vi "rsscope_core_global.vi"() -> ()   [LabVIEW 2018] (continued)
{"Level"=3, "Class Only"=FALSE, "Identifier"="RSSCOPE_ATTR_PROTOCOL_1000BASE_T1_REVERSE_DIFFERENTIAL_SOURCE", "Descriptive Name"="Protocol 1000BASE-T1 Reverse Differential Source", "Data Type"=0, "Command"="BUS{SerialBus}:TBTO:RDIF", "Access"=2, "Range Table"="rsscope_rngProtocolDataSource", "Read Callback"="", "Write Callback"="", "Supported Models"="", "Instrument Options"="K58", "Flags"=0, "Help"="Sets the source of the provided reversed differential signal, if RSSCOPE_ATTR_PROTOCOL_1000BASE_T1_REVERSE_SIGNAL_TYPE is set to differential.\n\nAvailable Repeated Capabilities:\nSerialBus: SB1, SB2, SB3, SB4\r\n\nRemote-control command(s):\nBUS<m>:TBTO:RDIF"}, {"Level"=3, "Class Only"=FALSE, "Identifier"="RSSCOPE_ATTR_PROTOCOL_1000BASE_T1_REVERSE_POSITIVE_SOURCE", "Descriptive Name"="Protocol 1000BASE-T1 Reverse Positive Source", "Data Type"=0, "Command"="BUS{SerialBus}:TBTO:RDAP", "Access"=2, "Range Table"="rsscope_rngProtocolDataSource", "Read Callback"="", "Write Callback"="", "Supported Models"="", "Instrument Options"="K58", "Flags"=0, "Help"="Selects the DA+ source of the provided reversed single ended signal, if RSSCOPE_ATTR_PROTOCOL_1000BASE_T1_REVERSE_SIGNAL_TYPE is set to single.\n\nAvailable Repeated Capabilities:\nSerialBus: SB1, SB2, SB3, SB4\r\n\nRemote-control command(s):\nBUS<m>:TBTO:RDAP"}, {"Level"=3, "Class Only"=FALSE, "Identifier"="RSSCOPE_ATTR_PROTOCOL_1000BASE_T1_REVERSE_NEGATIVE_SOURCE", "Descriptive Name"="Protocol 1000BASE-T1 Reverse Negative Source", "Data Type"=0, "Command"="BUS{SerialBus}:TBTO:RDAM", "Access"=2, "Range Table"="rsscope_rngProtocolDataSource", "Read Callback"="", "Write Callback"="", "Supported Models"="", "Instrument Options"="K58", "Flags"=0, "Help"="Selects the DA- source of the provided reversed single ended signal, if RSSCOPE_ATTR_PROTOCOL_1000BASE_T1_REVERSE_SIGNAL_TYPE is set to single.\n\nAvailable Repeated Capabilities:\nSerialBus: SB1, SB2, SB3, SB4\r\n\nRemote-control command(s):\nBUS<m>:TBTO:RDAM"}, {"Level"=3, "Class Only"=FALSE, "Identifier"="RSSCOPE_ATTR_PROTOCOL_1000BASE_T1_FORWARD_SIGNAL_TYPE", "Descriptive Name"="Protocol 1000BASE-T1 Forward Signal Type", "Data Type"=0, "Command"="BUS{SerialBus}:TBTO:FTYP", "Access"=2, "Range Table"="RsScope_rngSignalType", "Read Callback"="", "Write Callback"="", "Supported Models"="", "Instrument Options"="K58", "Flags"=0, "Help"="Sets the type of forward signal measurement.\n\nAvailable Repeated Capabilities:\nSerialBus: SB1, SB2, SB3, SB4\r\n\nRemote-control command(s):\nBUS<m>:TBTO:FTYP"}, {"Level"=3, "Class Only"=FALSE, "Identifier"="RSSCOPE_ATTR_PROTOCOL_1000BASE_T1_FORWARD_DIFFERENTIAL_SOURCE", "Descriptive Name"="Protocol 1000BASE-T1 Forward Differential Source", "Data Type"=0, "Command"="BUS{SerialBus}:TBTO:FDIF", "Access"=2, "Range Table"="rsscope_rngProtocolDataSource", "Read Callback"="", "Write Callback"="", "Supported Models"="", "Instrument Options"="K58", "Flags"=0, "Help"="Sets the source of the provided forward differential signal, if RSSCOPE_ATTR_PROTOCOL_1000BASE_T1_FORWARD_SIGNAL_TYPE is set to differential.\n\nAvailable Repeated Capabilities:\nSerialBus: SB1, SB2, SB3, SB4\r\n\nRemote-control command(s):\nBUS<m>:TBTO:FDIF"}, {"Level"=3, "Class Only"=FALSE, "Identifier"="RSSCOPE_ATTR_PROTOCOL_1000BASE_T1_FORWARD_POSITIVE_SOURCE", "Descriptive Name"="Protocol 1000BASE-T1 Forward Positive Source", "Data Type"=0, "Command"="BUS{SerialBus}:TBTO:FDAP", "Access"=2, "Range Table"="rsscope_rngProtocolDataSource", "Read Callback"="", "Write Callback"="", "Supported Models"="", "Instrument Options"="K58", "Flags"=0, "Help"="Selects the DA+ source of the provided forward single ended signal, if RSSCOPE_ATTR_PROTOCOL_1000BASE_T1_FORWARD_SIGNAL_TYPE is set to single.\n\nAvailable Repeated Capabilities:\nSerialBus: SB1, SB2, SB3, SB4\r\n\nRemote-control command(s):\nBUS<m>:TBTO:FDAP"}, {"Level"=3, "Class Only"=FALSE, "Identifier"="RSSCOPE_ATTR_PROTOCOL_1000BASE_T1_FORWARD_NEGATIVE_SOURCE", "Descriptive Name"="Protocol 1000BASE-T1 Forward Negative Source", "Data Type"=0, "Command"="BUS{SerialBus}:TBTO:FDAM", "Access"=2, "Range Table"="rsscope_rngProtocolDataSource", "Read Callback"="", "Write Callback"="", "Supported Models"="", "Instrument Options"="K58", "Flags"=0, "Help"="Selects the DA- source of the provided forward single ended signal, if RSSCOPE_ATTR_PROTOCOL_1000BASE_T1_FORWARD_SIGNAL_TYPE is set to single.\n\nAvailable Repeated Capabilities:\nSerialBus: SB1, SB2, SB3, SB4\r\n\nRemote-control command(s):\nBUS<m>:TBTO:FDAM"}, {"Level"=3, "Class Only"=FALSE, "Identifier"="RSSCOPE_ATTR_PROTOCOL_1000BASE_T1_ATTENUATION", "Descriptive Name"="Protocol 1000BASE-T1 Attenuation", "Data Type"=1, "Command"="BUS{SerialBus}:TBTO:ATTN", "Access"=2, "Range Table"="RsScope_rngProtocol1000BASE_T1Attenuation", "Read Callback"="", "Write Callback"="", "Supported Models"="", "Instrument Options"="K58", "Flags"=0, "Help"="Sets the attenuation factor. It is used to de-amplify the reverse signal before subtracting it from the forward signal.\n\nAvailable Repeated Capabilities:\nSerialBus: SB1, SB2, SB3, SB4\r\n\nRemote-control command(s):\nBUS<m>:TBTO:ATTN"}, {"Level"=3, "Class Only"=FALSE, "Identifier"="RSSCOPE_ATTR_PROTOCOL_1000BASE_T1_POLARITY", "Descriptive Name"="Protocol 1000BASE-T1 Polarity", "Data Type"=0, "Command"="BUS{SerialBus}:TBTO:POL", "Access"=2, "Range Table"="rsscope_rngEthernetPolarity", "Read Callback"="", "Write Callback"="", "Supported Models"="", "Instrument Options"="K58", "Flags"=0, "Help"="Selects the polarity of the data signal.\n\nAvailable Repeated Capabilities:\nSerialBus: SB1, SB2, SB3, SB4\r\n\nRemote-control command(s):\nBUS<m>:TBTO:POLarity"}, {"Level"=3, "Class Only"=FALSE, "Identifier"="RSSCOPE_ATTR_PROTOCOL_1000BASE_T1_MODE", "Descriptive Name"="Protocol 1000BASE-T1 Mode", "Data Type"=0, "Command"="BUS{SerialBus}:TBTO:MODE", "Access"=2, "Range Table"="RsScope_rngSignalDirection", "Read Callback"="", "Write Callback"="", "Supported Models"="", "Instrument Options"="K58", "Flags"=0, "Help"="Selects the direction of the full-duplex signal you want to look at.\n\nAvailable Repeated Capabilities:\nSerialBus: SB1, SB2, SB3, SB4\r\n\nRemote-control command(s):\nBUS<m>:TBTO:MODE"}, {"Level"=3, "Class Only"=FALSE, "Identifier"="RSSCOPE_ATTR_PROTOCOL_1000BASE_T1_SYMBOL_RATE", "Descriptive Name"="Protocol 1000BASE-T1 Symbol Rate", "Data Type"=1, "Command"="BUS{SerialBus}:TBTO:SYMR", "Access"=2, "Range Table"="RsScope_rngProtocol1000BASE_T1SymbolRate", "Read Callback"="", "Write Callback"="", "Supported Models"="", "Instrument Options"="K58", "Flags"=0, "Help"="Defines the rate of ternary symbols.\n\nAvailable Repeated Capabilities:\nSerialBus: SB1, SB2, SB3, SB4\r\n\nRemote-control command(s):\nBUS<m>:TBTO:SYMRate"}, {"Level"=3, "Class Only"=TRUE, "Identifier"="", "Descriptive Name"="Decoding Results", "Data Type"=0, "Command"="", "Access"=0, "Range Table"="", "Read Callback"="", "Write Callback"="", "Supported Models"="", "Instrument Options"="", "Flags"=0, "Help"="Returns the 1000BASE-T1 decoding results."}, {"Level"=4, "Class Only"=FALSE, "Identifier"="RSSCOPE_ATTR_PROTOCOL_1000BASE_T1_FRAME_COUNT", "Descriptive Name"="Protocol 1000BASE-T1 Frame Count", "Data Type"=0, "Command"="BUS{SerialBus}:TBTO:RES:FCO?", "Access"=0, "Range Table"="", "Read Callback"="", "Write Callback"="", "Supported Models"="", "Instrument Options"="K58", "Flags"=0, "Help"="Returns the number of decoded frames.\n\nAvailable Repeated Capabilities:\nSerialBus: SB1, SB2, SB3, SB4\r\n\nRemote-control command(s):\nBUS<m>:TBTO:RESult:FCOunt?"}, {"Level"=4, "Class Only"=FALSE, "Identifier"="RSSCOPE_ATTR_PROTOCOL_1000BASE_T1_SELECTED_FRAME", "Descriptive Name"="Protocol 1000BASE-T1 Selected Frame", "Data Type"=0, "Command"="", "Access"=2, "Range Table"="", "Read Callback"="", "Write Callback"="", "Supported Models"="", "Instrument Options"="K58", "Flags"=0, "Help"="Sets the selector for the Frame repeated capability.\n\nAvailable Repeated Capabilities:\nNone\n\nRemote-control command(s):\n"}, {"Level"=4, "Class Only"=FALSE, "Identifier"="RSSCOPE_ATTR_PROTOCOL_1000BASE_T1_FRAME_STATUS", "Descriptive Name"="Protocol 1000BASE-T1 Frame Status", "Data Type"=0, "Command"="BUS{SerialBus}:TBTO:RES:FRAM<Frame>:STAT?", "Access"=0, "Range Table"="RsScope_rngProtocol1000BASE_T1FrameStatus", "Read Callback"="rsscope_Format1000BASE_T1FrameRepCapInt32_ReadCallback.vi", "Write Callback"="", "Supported Models"="", "Instrument Options"="K58", "Flags"=0, "Help"="Returns the state of the frame.\n\nAvailable Repeated Capabilities:\nSerialBus: SB1, SB2, SB3, SB4\r\n\nRemote-control command(s):\nBUS<m>:TBTO:RESult:FRAMe<n>:STATe?"}, {"Level"=4, "Class Only"=FALSE, "Identifier"="RSSCOPE_ATTR_PROTOCOL_1000BASE_T1_FRAME_START_TIME", "Descriptive Name"="Protocol 1000BASE-T1 Frame Start Time", "Data Type"=1, "Command"="BUS{SerialBus}:TBTO:RES:FRAM<Frame>:STAR?", "Access"=0, "Range Table"="", "Read Callback"="rsscope_Format1000BASE_T1FrameRepCapReal64_ReadCallback.vi", "Write Callback"="", "Supported Models"="", "Instrument Options"="K58", "Flags"=0, "Help"="Returns the start time of the selected frame.\n\nAvailable Repeated Capabilities:\nSerialBus: SB1, SB2, SB3, SB4\r\n\nRemote-control command(s):\nBUS<m>:TBTO:RESult:FRAMe<n>:STARt?"}, {"Level"=4, "Class Only"=FALSE, "Identifier"="RSSCOPE_ATTR_PROTOCOL_1000BASE_T1_FRAME_STOP_TIME", "Descriptive Name"="Protocol 1000BASE-T1 Frame Stop Time", "Data Type"=1, "Command"="BUS{SerialBus}:TBTO:RES:FRAM<Frame>:STOP?", "Access"=0, "Range Table"="", "Read Callback"="rsscope_Format1000BASE_T1FrameRepCapReal64_ReadCallback.vi", "Write Callback"="", "Supported Models"="", "Instrument Options"="K58", "Flags"=0, "Help"="Returns the end time of the selected frame.\n\nAvailable Repeated Capabilities:\nSerialBus: SB1, SB2, SB3, SB4\r\n\nRemote-control command(s):\nBUS<m>:TBTO:RESult:FRAMe<n>:STOP?"}, {"Level"=4, "Class Only"=FALSE, "Identifier"="RSSCOPE_ATTR_PROTOCOL_1000BASE_T1_FRAME_LENGTH", "Descriptive Name"="Protocol 1000BASE-T1 Frame Length", "Data Type"=0, "Command"="BUS{SerialBus}:TBTO:RES:FRAM<Frame>:TYPE?", "Access"=0, "Range Table"="", "Read Callback"="rsscope_Format1000BASE_T1FrameRepCapInt32_ReadCallback.vi", "Write Callback"="", "Supported Models"="", "Instrument Options"="K58", "Flags"=0, "Help"="Returns the value of length / type field of the selected frame.\n\nAvailable Repeated Capabilities:\nSerialBus: SB1, SB2, SB3, SB4\r\n\nRemote-control command(s):\nBUS<m>:TBTO:RESult:FRAMe<n>:TYPE?"}, {"Level"=4, "Class Only"=FALSE, "Identifier"="RSSCOPE_ATTR_PROTOCOL_1000BASE_T1_FRAME_CRC", "Descriptive Name"="Protocol 1000BASE-T1 Frame CRC", "Data Type"=5, "Command"="BUS{SerialBus}:TBTO:RES:FRAM<Frame>:CRC?", "Access"=0, "Range Table"="", "Read Callback"="rsscope_Format1000BASE_T1FrameRepCapInt64_ReadCallback.vi", "Write Callback"="", "Supported Models"="", "Instrument Options"="K58", "Flags"=0, "Help"="Returns the CRC (frame check) checksum of the selected frame.\n\nAvailable Repeated Capabilities:\nSerialBus: SB1, SB2, SB3, SB4\r\n\nRemote-control command(s):\nBUS<m>:TBTO:RESult:FRAMe<n>:CRC?"}, {"Level"=4, "Class Only"=FALSE, "Identifier"="RSSCOPE_ATTR_PROTOCOL_1000BASE_T1_FRAME_DATA_BYTES_RAWSTRING", "Descriptive Name"="Protocol 1000BASE-T1 Frame Data Bytes RawString", "Data Type"=6, "Command"="BUS{SerialBus}:TBTO:RES:FRAM<Frame>:DATA?", "Access"=0, "Range Table"="", "Read Callback"="rsscope_Format1000BASE_T1FrameRepCapString_ReadCallback.vi", "Write Callback"="", "Supported Models"="", "Instrument Options"="K58", "Flags"=0, "Help"="Returns the data for the selected frame.\n\nAvailable Repeated Capabilities:\nSerialBus: SB1, SB2, SB3, SB4\r\n\nRemote-control command(s):\nBUS<m>:TBTO:RESult:FRAMe<n>:DATA?"}, {"Level"=4, "Class Only"=FALSE, "Identifier"="RSSCOPE_ATTR_PROTOCOL_1000BASE_T1_FRAME_DESTINATION", "Descriptive Name"="Protocol 1000BASE-T1 Frame Destination", "Data Type"=2, "Command"="BUS{SerialBus}:TBTO:RES:FRAM<Frame>:DEST?", "Access"=0, "Range Table"="", "Read Callback"="rsscope_Format1000BASE_T1FrameRepCapString_ReadCallback.vi", "Write Callback"="", "Supported Models"="", "Instrument Options"="K58", "Flags"=0, "Help"="Returns the destination address of the selected frame.\n\nAvailable Repeated Capabilities:\nSerialBus: SB1, SB2, SB3, SB4\r\n\nRemote-control command(s):\nBUS<m>:TBTO:RESult:FRAMe<n>:DESTaddress?"}, {"Level"=4, "Class Only"=FALSE, "Identifier"="RSSCOPE_ATTR_PROTOCOL_1000BASE_T1_FRAME_DESTINATION_SYMBOLS", "Descriptive Name"="Protocol 1000BASE-T1 Frame Destination Symbols", "Data Type"=2, "Command"="BUS{SerialBus}:TBTO:RES:FRAM<Frame>:DSYM?", "Access"=0, "Range Table"="", "Read Callback"="rsscope_Format1000BASE_T1FrameRepCapString_ReadCallback.vi", "Write Callback"="", "Supported Models"="", "Instrument Options"="K58", "Flags"=0, "Help"="Returns the destination symbols of the selected frame.\n\nAvailable Repeated Capabilities:\nSerialBus: SB1, SB2, SB3, SB4\r\n\nRemote-control command(s):\nBUS<m>:TBTO:RESult:FRAMe<n>:DSYMbol?"}, {"Level"=4, "Class Only"=FALSE, "Identifier"="RSSCOPE_ATTR_PROTOCOL_1000BASE_T1_FRAME_SOURCE", "Descriptive Name"="Protocol 1000BASE-T1 Frame Source", "Data Type"=2, "Command"="BUS{SerialBus}:TBTO:RES:FRAM<Frame>:SRC?", "Access"=0, "Range Table"="", "Read Callback"="rsscope_Format1000BASE_T1FrameRepCapString_ReadCallback.vi", "Write Callback"="", "Supported Models"="", "Instrument Options"="K58", "Flags"=0, "Help"="Returns the source address of the selected frame.\n\nAvailable Repeated Capabilities:\nSerialBus: SB1, SB2, SB3, SB4\r\n\nRemote-control command(s):\nBUS<m>:TBTO:RESult:FRAMe<n>:SRCaddress?"}, {"Level"=4, "Class Only"=FALSE, "Identifier"="RSSCOPE_ATTR_PROTOCOL_1000BASE_T1_FRAME_SOURCE_SYMBOLS", "Descriptive Name"="Protocol 1000BASE-T1 Frame Source Symbols", "Data Type"=2, "Command"="BUS{SerialBus}:TBTO:RES:FRAM<Frame>:SSYM?", "Access"=0, "Range Table"="", "Read Callback"="rsscope_Format1000BASE_T1FrameRepCapString_ReadCallback.vi", "Write Callback"="", "Supported Models"="", "Instrument Options"="K58", "Flags"=0, "Help"="Returns the source symbols of the selected frame.\n\nAvailable Repeated Capabilities:\nSerialBus: SB1, SB2, SB3, SB4\r\n\nRemote-control command(s):\nBUS<m>:TBTO:RESult:FRAMe<n>:SSYMbol?"}, {"Level"=4, "Class Only"=FALSE, "Identifier"="RSSCOPE_ATTR_PROTOCOL_1000BASE_T1_FRAME_BIT_RATE", "Descriptive Name"="Protocol 1000BASE-T1 Frame Bit Rate", "Data Type"=5, "Command"="BUS{SerialBus}:TBTO:RES:FRAM<Frame>:BITR?", "Access"=0, "Range Table"="", "Read Callback"="rsscope_Format1000BASE_T1FrameRepCapInt64_ReadCallback.vi", "Write Callback"="", "Supported Models"="", "Instrument Options"="K58", "Flags"=0, "Help"="Returns the primary bit rate.\n\nAvailable Repeated Capabilities:\nSerialBus: SB1, SB2, SB3, SB4\r\n\nRemote-control command(s):\nBUS<m>:TBTO:RESult:FRAMe<n>:BITRate?"}, {"Level"=4, "Class Only"=FALSE, "Identifier"="RSSCOPE_ATTR_PROTOCOL_1000BASE_T1_FRAME_TYPE", "Descriptive Name"="Protocol 1000BASE-T1 Frame Type", "Data Type"=0, "Command"="BUS{SerialBus}:TBTO:RES:FRAM<Frame>:FTYP?", "Access"=0, "Range Table"="RsScope_rngProtocol1000BASE_T1FrameType", "Read Callback"="rsscope_Format1000BASE_T1FrameRepCapInt32_ReadCallback.vi", "Write Callback"="", "Supported Models"="", "Instrument Options"="K58", "Flags"=0, "Help"="Returns the type of the selected frame.\n\nAvailable Repeated Capabilities:\nSerialBus: SB1, SB2, SB3, SB4\r\n\nRemote-control command(s):\nBUS<m>:TBTO:RESult:FRAMe<n>:FTYPe?"}, {"Level"=4, "Class Only"=FALSE, "Identifier"="RSSCOPE_ATTR_PROTOCOL_1000BASE_T1_FRAME_NUMBER_OF_WORDS", "Descriptive Name"="Protocol 1000BASE-T1 Frame Number Of Words", "Data Type"=5, "Command"="BUS{SerialBus}:TBTO:RES:FRAM<Frame>:NUMW?", "Access"=0, "Range Table"="", "Read Callback"="rsscope_Format1000BASE_T1FrameRepCapInt64_ReadCallback.vi", "Write Callback"="", "Supported Models"="", "Instrument Options"="K58", "Flags"=0, "Help"="Returns the number of decoded words for the selected frame.\n\nAvailable Repeated Capabilities:\nSerialBus: SB1, SB2, SB3, SB4\r\n\nRemote-control command(s):\nBUS<m>:TBTO:RESult:FRAMe<n>:NUMWords?"}, {"Level"=4, "Class Only"=FALSE, "Identifier"="RSSCOPE_ATTR_PROTOCOL_1000BASE_T1_SELECTED_WORD", "Descriptive Name"="Protocol 1000BASE-T1 Selected Word", "Data Type"=5, "Command"="", "Access"=2, "Range Table"="", "Read Callback"="", "Write Callback"="", "Supported Models"="", "Instrument Options"="K58", "Flags"=0, "Help"="Sets the selector for the Word repeated capability.\n\nAvailable Repeated Capabilities:\nNone\n\nRemote-control command(s):\n"}, {"Level"=4, "Class Only"=FALSE, "Identifier"="RSSCOPE_ATTR_PROTOCOL_1000BASE_T1_FRAME_WORD_TYPE", "Descriptive Name"="Protocol 1000BASE-T1 Frame Word Type", "Data Type"=2, "Command"="BUS{SerialBus}:TBTO:RES:FRAM<Frame>:WORD<Word>:TYPE?", "Access"=0, "Range Table"="", "Read Callback"="rsscope_Format1000BASE_T1WordRepCapString_ReadCallback.vi", "Write Callback"="", "Supported Models"="", "Instrument Options"="K58", "Flags"=0, "Help"="Returns the data type for the selected word.\n\nAvailable Repeated Capabilities:\nSerialBus: SB1, SB2, SB3, SB4\r\n\nRemote-control command(s):\nBUS<m>:TBTO:RESult:FRAMe<n>:WORD<o>:TYPE?"}, {"Level"=4, "Class Only"=FALSE, "Identifier"="RSSCOPE_ATTR_PROTOCOL_1000BASE_T1_FRAME_WORD_VALUE", "Descriptive Name"="Protocol 1000BASE-T1 Frame Word Value", "Data Type"=0, "Command"="BUS{SerialBus}:TBTO:RES:FRAM<Frame>:WORD<Word>:VAL?", "Access"=0, "Range Table"="", "Read Callback"="rsscope_Format1000BASE_T1WordRepCapInt32_ReadCallback.vi", "Write Callback"="", "Supported Models"="", "Instrument Options"="K58", "Flags"=0, "Help"="Returns the data value for the selected word.\n\nAvailable Repeated Capabilities:\nSerialBus: SB1, SB2, SB3, SB4\r\n\nRemote-control command(s):\nBUS<m>:TBTO:RESult:FRAMe<n>:WORD<o>:VALue?"}, {"Level"=1, "Class Only"=TRUE, "Identifier"="", "Descriptive Name"="Power Analysis", "Data Type"=0, "Command"="", "Access"=0, "Range Table"="", "Read Callback"="", "Write Callback"="", "Supported Models"="", "Instrument Options"="", "Flags"=0, "Help"="Power Analysis"}, {"Level"=2, "Class Only"=FALSE, "Identifier"="RSSCOPE_ATTR_POWER_ANALYSIS_MODE", "Descriptive Name"="Power Analysis Mode", "Data Type"=4, "Command"="POW:ENAB", "Access"=1, "Range Table"="", "Read Callback"="", "Write Callback"="", "Supported Models"="", "Instrument Options"="", "Flags"=0, "Help"="Activates the power analysis measurement.\n\nAvailable Repeated Capabilities:\nNone\n\nRemote-control command(s):\nPOWer:ENABle"}, {"Level"=2, "Class Only"=TRUE, "Identifier"="", "Descriptive Name"="Source", "Data Type"=0, "Command"="", "Access"=0, "Range Table"="", "Read Callback"="", "Write Callback"="", "Supported Models"="", "Instrument Options"="", "Flags"=0, "Help"="Class for attributes with SourceNumber repcap."}, {"Level"=3, "Class Only"=FALSE, "Identifier"="RSSCOPE_ATTR_POWER_ANALYSIS_VOLTAGE_SOURCE", "Descriptive Name"="Power Analysis Voltage Source", "Data Type"=0, "Command"="POW:SOUR:VOLT{SourceNumber}", "Access"=2, "Range Table"="RsScope_rngPowerAnalysisSource", "Read Callback"="", "Write Callback"="", "Supported Models"="", "Instrument Options"="", "Flags"=0, "Help"="Sets the channel for the voltage source input.\n\nAvailable Repeated Capabilities:\nSourceNumber: SN1, SN2, SN3, SN4\r\n\nRemote-control command(s):\nPOWer:SOURce:VOLTage<1..4>"}, {"Level"=3, "Class Only"=FALSE, "Identifier"="RSSCOPE_ATTR_POWER_ANALYSIS_CURRENT_SOURCE", "Descriptive Name"="Power Analysis Current Source", "Data Type"=0, "Command"="POW:SOUR:CURR{SourceNumber}", "Access"=2, "Range Table"="RsScope_rngPowerAnalysisSource", "Read Callback"="", "Write Callback"="", "Supported Models"="", "Instrument Options"="", "Flags"=0, "Help"="Sets the channel for the current source input.\n\nAvailable Repeated Capabilities:\nSourceNumber: SN1, SN2, SN3, SN4\r\n\nRemote-control command(s):\nPOWer:SOURce:CURRent<1..2>"}, {"Level"=2, "Class Only"=TRUE, "Identifier"="", "Descriptive Name"="Deskew", "Data Type"=0, "Command"="", "Access"=0, "Range Table"="", "Read Callback"="", "Write Callback"="", "Supported Models"="", "Instrument Options"="", "Flags"=0, "Help"="Deskew of the current and voltage probes"}, {"Level"=3, "Class Only"=FALSE, "Identifier"="RSSCOPE_ATTR_POWER_ANALYSIS_START_DESKEW", "Descriptive Name"="Power Analysis Start Deskew", "Data Type"=4, "Command"="POW:DESK:EXEC;*WAI", "Access"=1, "Range Table"="", "Read Callback"="", "Write Callback"="", "Supported Models"="", "Instrument Options"="", "Flags"=0, "Help"="Starts the auto deskew.\n\nAvailable Repeated Capabilities:\nNone\n\nRemote-control command(s):\nPOWer:DESKew:EXECute"}, {"Level"=3, "Class Only"=FALSE, "Identifier"="RSSCOPE_ATTR_POWER_ANALYSIS_DESKEW_RESET", "Descriptive Name"="Power Analysis Deskew Reset", "Data Type"=3, "Command"="POW:DESK:RES", "Access"=2, "Range Table"="", "Read Callback"="", "Write Callback"="", "Supported Models"="", "Instrument Options"="", "Flags"=0, "Help"="Overwrites the present skew setup.\n\nAvailable Repeated Capabilities:\nNone\n\nRemote-control command(s):\nPOWer:DESKew:RESet"}, {"Level"=3, "Class Only"=FALSE, "Identifier"="RSSCOPE_ATTR_POWER_ANALYSIS_DESKEW_TIME", "Descriptive Name"="Power Analysis Deskew Time", "Data Type"=1, "Command"="POW:DESK:TIME?", "Access"=0, "Range Table"="", "Read Callback"="", "Write Callback"="", "Supported Models"="", "Instrument Options"="", "Flags"=0, "Help"="Queries the result of the auto deskew.\n\nAvailable Repeated Capabilities:\nNone\n\nRemote-control command(s):\nPOWer:DESKew:TIME?"}, {"Level"=3, "Class Only"=FALSE, "Identifier"="RSSCOPE_ATTR_POWER_ANALYSIS_DESKEW_CURRENT", "Descriptive Name"="Power Analysis Deskew Current", "Data Type"=4, "Command"="POW:DESK:CURR", "Access"=1, "Range Table"="", "Read Callback"="", "Write Callback"="", "Supported Models"="", "Instrument Options"="", "Flags"=0, "Help"="Applies the result of the auto deskew to the &apos;Skew offset&apos; value.\n\nAvailable Repeated Capabilities:\nNone\n\nRemote-control command(s):\nPOWer:DESKew:CURRent"}, {"Level"=3, "Class Only"=FALSE, "Identifier"="RSSCOPE_ATTR_POWER_ANALYSIS_DESKEW_USER_DEFINED_RESET", "Descriptive Name"="Power Analysis Deskew User Defined Reset", "Data Type"=3, "Command"="POW:DESK:UDPR", "Access"=2, "Range Table"="", "Read Callback"="", "Write Callback"="", "Supported Models"="", "Instrument Options"="", "Flags"=0, "Help"="Activates or deactivates a user defined setup. If ON, the instrument setup including probe setup and the deskew values are written to a user defined preset file (saveset) that can be loaded using MMEMory:RCL\n\nAvailable Repeated Capabilities:\nNone\n\nRemote-control command(s):\nPOWer:DESKew:UDPReset"}, {"Level"=3, "Class Only"=TRUE, "Identifier"="", "Descriptive Name"="Channel", "Data Type"=0, "Command"="", "Access"=0, "Range Table"="", "Read Callback"="", "Write Callback"="", "Supported Models"="", "Instrument Options"="", "Flags"=0, "Help"="Commands depended on channel number (repeated capability Channel)"}, {"Level"=4, "Class Only"=FALSE, "Identifier"="RSSCOPE_ATTR_POWER_ANALYSE_PROBE_MODE", "Descriptive Name"="Power Analyse Probe Mode", "Data Type"=0, "Command"="PROB{Channel}:SET:DISP", "Access"=2, "Range Table"="RsScope_rngPowerAnalyseProbeMode", "Read Callback"="", "Write Callback"="", "Supported Models"="", "Instrument Options"="", "Flags"=0, "Help"="Selects the input voltages to be measured by the Probe Meter of an R&S differential active probe.\n\nAvailable Repeated Capabilities:\nChannel: CH1, CH2, CH3, CH4, CHExt\r\n\nRemote-control command(s):\nPROBe<m>:SETup:DISPlaydiff"}, {"Level"=2, "Class Only"=TRUE, "Identifier"="", "Descriptive Name"="DUT", "Data Type"=0, "Command"="", "Access"=0, "Range Table"="", "Read Callback"="", "Write Callback"="", "Supported Models"="", "Instrument Options"="", "Flags"=0, "Help"="Characterizes your device under test (DUT)."}, {"Level"=3, "Class Only"=FALSE, "Identifier"="RSSCOPE_ATTR_POWER_ANALYSIS_DUT_NAME", "Descriptive Name"="Power Analysis DUT Name", "Data Type"=2, "Command"="POW:REP:DUT", "Access"=2, "Range Table"="", "Read Callback"="", "Write Callback"="", "Supported Models"="", "Instrument Options"="", "Flags"=0, "Help"="Enter a name for your DUT.\n\nAvailable Repeated Capabilities:\nNone\n\nRemote-control command(s):\nPOWer:REPort:DUT"}, {"Level"=3, "Class Only"=FALSE, "Identifier"="RSSCOPE_ATTR_POWER_ANALYSIS_USER", "Descriptive Name"="Power Analysis User", "Data Type"=2, "Command"="POW:REP:USER", "Access"=2, "Range Table"="", "Read Callback"="", "Write Callback"="", "Supported Models"="", "Instrument Options"="", "Flags"=0, "Help"="Enter a user.\n\nAvailable Repeated Capabilities:\nNone\n\nRemote-control command(s):\nPOWer:REPort:USER"}, {"Level"=3, "Class Only"=FALSE, "Identifier"="RSSCOPE_ATTR_POWER_ANALYSIS_SITE", "Descriptive Name"="Power Analysis Site", "Data Type"=2, "Command"="POW:REP:SITE", "Access"=2, "Range Table"="", "Read Callback"="", "Write Callback"="", "Supported Models"="", "Instrument Options"="", "Flags"=0, "Help"="Enter a site.\n\nAvailable Repeated Capabilities:\nNone\n\nRemote-control command(s):\nPOWer:REPort:SITE"}, {"Level"=3, "Class Only"=FALSE, "Identifier"="RSSCOPE_ATTR_POWER_ANALYSIS_TEMPERATURE", "Descriptive Name"="Power Analysis Temperature", "Data Type"=0, "Command"="POW:REP:TEMP", "Access"=2, "Range Table"="", "Read Callback"="", "Write Callback"="", "Supported Models"="", "Instrument Options"="", "Flags"=0, "Help"="Enter a temperature.\n\nAvailable Repeated Capabilities:\nNone\n\nRemote-control command(s):\nPOWer:REPort:TEMPerature"}, {"Level"=3, "Class Only"=FALSE, "Identifier"="RSSCOPE_ATTR_POWER_ANALYSIS_DESCRIPTION", "Descriptive Name"="Power Analysis Description", "Data Type"=2, "Command"="POW:REP:DESC", "Access"=2, "Range Table"="", "Read Callback"="", "Write Callback"="", "Supported Models"="", "Instrument Options"="", "Flags"=0, "Help"="Enter a description.\n\nAvailable Repeated Capabilities:\nNone\n\nRemote-control command(s):\nPOWer:REPort:DESCription"}, {"Level"=2, "Class Only"=TRUE, "Identifier"="", "Descriptive Name"="Report", "Data Type"=0, "Command"="", "Access"=0, "Range Table"="", "Read Callback"="", "Write Callback"="", "Supported Models"="", "Instrument Options"="", "Flags"=0, "Help"="Power Measurement Reports"}, {"Level"=3, "Class Only"=FALSE, "Identifier"="RSSCOPE_ATTR_POWER_ANALYSIS_REPORT_ADD", "Descriptive Name"="Power Analysis Report Add", "Data Type"=0, "Command"="POW:REP:TEST:ADD", "Access"=1, "Range Table"="RsScope_rngPowerAnalysisMeasurementType", "Read Callback"="", "Write Callback"="", "Supported Models"="", "Instrument Options"="", "Flags"=0, "Help"="Adds the selected measurement to the report.\n\nAvailable Repeated Capabilities:\nNone\n\nRemote-control command(s):\nPOWer:REPort:TEST:ADD"}, {"Level"=3, "Class Only"=FALSE, "Identifier"="RSSCOPE_ATTR_POWER_ANALYSIS_REPORT_SEL_ALL", "Descriptive Name"="Power Analysis Report Select All", "Data Type"=0, "Command"="POW:REP:TEST:SEA", "Access"=1, "Range Table"="RsScope_rngPowerAnalysisMeasurementType", "Read Callback"="", "Write Callback"="", "Supported Models"="", "Instrument Options"="", "Flags"=0, "Help"="Selects all result reports.\n\nAvailable Repeated Capabilities:\nNone\n\nRemote-control command(s):\nPOWer:REPort:TEST:SEA"}, {"Level"=3, "Class Only"=FALSE, "Identifier"="RSSCOPE_ATTR_POWER_ANALYSIS_REPORT_SEL_NONE", "Descriptive Name"="Power Analysis Report Deselect All", "Data Type"=0, "Command"="POW:REP:TEST:DSEA", "Access"=1, "Range Table"="RsScope_rngPowerAnalysisMeasurementType", "Read Callback"="", "Write Callback"="", "Supported Models"="", "Instrument Options"="", "Flags"=0, "Help"="Deselects all result reports.\n\nAvailable Repeated Capabilities:\nNone\n\nRemote-control command(s):\nPOWer:REPort:TEST:DSEA"}, {"Level"=3, "Class Only"=FALSE, "Identifier"="RSSCOPE_ATTR_POWER_ANALYSIS_REPORT_SEL_REMOVE", "Descriptive Name"="Power Analysis Report Remove Selected", "Data Type"=0, "Command"="POW:REP:TEST:RSE", "Access"=1, "Range Table"="RsScope_rngPowerAnalysisMeasurementType", "Read Callback"="", "Write Callback"="", "Supported Models"="", "Instrument Options"="", "Flags"=0, "Help"="Removes the selected result report.\n\nAvailable Repeated Capabilities:\nNone\n\nRemote-control command(s):\nPOWer:REPort:TEST:RSE"}, {"Level"=3, "Class Only"=FALSE, "Identifier"="RSSCOPE_ATTR_POWER_ANALYSIS_REPORT_SEL_INVERT", "Descriptive Name"="Power Analysis Report Invert Selection", "Data Type"=0, "Command"="POW:REP:TEST:ISE", "Access"=1, "Range Table"="RsScope_rngPowerAnalysisMeasurementType", "Read Callback"="", "Write Callback"="", "Supported Models"="", "Instrument Options"="", "Flags"=0, "Help"="Inverts the selection of all result reports, meaning that all selected result reports are deselected and vice versa.\n\nAvailable Repeated Capabilities:\nNone\n\nRemote-control command(s):\nPOWer:REPort:TEST:ISE"}, {"Level"=3, "Class Only"=FALSE, "Identifier"="RSSCOPE_ATTR_POWER_ANALYSIS_REPORT_FILE_NEW", "Descriptive Name"="Power Analysis Report File New", "Data Type"=4, "Command"="POW:REP:FILE:NEW", "Access"=1, "Range Table"="", "Read Callback"="", "Write Callback"="", "Supported Models"="", "Instrument Options"="", "Flags"=0, "Help"="Creates new file.\n\nAvailable Repeated Capabilities:\nNone\n\nRemote-control command(s):\nPOWer:REPort:FILE:NEW"}, {"Level"=3, "Class Only"=FALSE, "Identifier"="RSSCOPE_ATTR_POWER_ANALYSIS_REPORT_FILE_NAME", "Descriptive Name"="Power Analysis Report File Name", "Data Type"=2, "Command"="POW:REP:FILE:NAME", "Access"=1, "Range Table"="", "Read Callback"="", "Write Callback"="", "Supported Models"="", "Instrument Options"="", "Flags"=0, "Help"="Renames the file\n\nAvailable Repeated Capabilities:\nNone\n\nRemote-control command(s):\nPOWer:REPort:FILE:NAME"}, {"Level"=3, "Class Only"=FALSE, "Identifier"="RSSCOPE_ATTR_POWER_ANALYSIS_REPORT_FILE_SAVE", "Descriptive Name"="Power Analysis Report File Save", "Data Type"=4, "Command"="POW:REP:FILE:SAVE", "Access"=1, "Range Table"="", "Read Callback"="", "Write Callback"="", "Supported Models"="", "Instrument Options"="", "Flags"=0, "Help"="Saves the file\n\nAvailable Repeated Capabilities:\nNone\n\nRemote-control command(s):\nPOWer:REPort:FILE:SAVE"}, {"Level"=3, "Class Only"=FALSE, "Identifier"="RSSCOPE_ATTR_POWER_ANALYSIS_REPORT_FILE_DELETE", "Descriptive Name"="Power Analysis Report File Delete", "Data Type"=4, "Command"="POW:REP:FILE:DEL", "Access"=1, "Range Table"="", "Read Callback"="", "Write Callback"="", "Supported Models"="", "Instrument Options"="", "Flags"=0, "Help"="Deletes the selected file\n\nAvailable Repeated Capabilities:\nNone\n\nRemote-control command(s):\nPOWer:REPort:FILE:DELete"}, {"Level"=3, "Class Only"=TRUE, "Identifier"="", "Descriptive Name"="Layout", "Data Type"=0, "Command"="", "Access"=0, "Range Table"="", "Read Callback"="", "Write Callback"="", "Supported Models"="", "Instrument Options"="", "Flags"=0, "Help"="Sets a layout for your report."}, {"Level"=4, "Class Only"=FALSE, "Identifier"="RSSCOPE_ATTR_POWER_ANALYSIS_REPORT_PAPER_SIZE", "Descriptive Name"="Power Analysis Report Paper Size", "Data Type"=0, "Command"="POW:REP:PAP", "Access"=2, "Range Table"="RsScope_rngPowerAnalysisReportPaperSize", "Read Callback"="", "Write Callback"="", "Supported Models"="", "Instrument Options"="", "Flags"=0, "Help"="Sets the paper size.\n\nAvailable Repeated Capabilities:\nNone\n\nRemote-control command(s):\nPOWer:REPort:PAPersize"}, {"Level"=4, "Class Only"=FALSE, "Identifier"="RSSCOPE_ATTR_POWER_ANALYSIS_REPORT_FONT", "Descriptive Name"="Power Analysis Report Font", "Data Type"=0, "Command"="POW:REP:FONT:FAMI", "Access"=2, "Range Table"="RsScope_rngPowerAnalysisReportFont", "Read Callback"="", "Write Callback"="", "Supported Models"="", "Instrument Options"="", "Flags"=0, "Help"="Selects the font family.\n\nAvailable Repeated Capabilities:\nNone\n\nRemote-control command(s):\nPOWer:REPort:FONT:FAMI"}, {"Level"=4, "Class Only"=FALSE, "Identifier"="RSSCOPE_ATTR_POWER_ANALYSIS_REPORT_FONT_SIZE", "Descriptive Name"="Power Analysis Report Font Size", "Data Type"=0, "Command"="POW:REP:FONT:SIZE", "Access"=2, "Range Table"="RsScope_rngPowerAnalysisReportFontSize", "Read Callback"="", "Write Callback"="", "Supported Models"="", "Instrument Options"="", "Flags"=0, "Help"="Selects the font size.\n\nAvailable Repeated Capabilities:\nNone\n\nRemote-control command(s):\nPOWer:REPort:FONT:SIZE"}, {"Level"=4, "Class Only"=FALSE, "Identifier"="RSSCOPE_ATTR_POWER_ANALYSIS_REPORT_FONT_COLOR", "Descriptive Name"="Power Analysis Report Font Color", "Data Type"=0, "Command"="POW:REP:FONT:COLO", "Access"=2, "Range Table"="", "Read Callback"="", "Write Callback"="", "Supported Models"="", "Instrument Options"="", "Flags"=0, "Help"="Selects the font color.\n\nAvailable Repeated Capabilities:\nNone\n\nRemote-control command(s):\nPOWer:REPort:FONT:COLO"}, {"Level"=4, "Class Only"=FALSE, "Identifier"="RSSCOPE_ATTR_POWER_ANALYSIS_REPORT_LOGO", "Descriptive Name"="Power Analysis Report Logo", "Data Type"=2, "Command"="POW:REP:LOGO", "Access"=2, "Range Table"="", "Read Callback"="", "Write Callback"="", "Supported Models"="", "Instrument Options"="", "Flags"=0, "Help"="Selects a path to a logo picture file.\n\nAvailable Repeated Capabilities:\nNone\n\nRemote-control command(s):\nPOWer:REPort:LOGO"}, {"Level"=4, "Class Only"=FALSE, "Identifier"="RSSCOPE_ATTR_POWER_ANALYSIS_REPORT_INV_COLOR", "Descriptive Name"="Power Analysis Report Invert Scr Color", "Data Type"=3, "Command"="POW:REP:INV", "Access"=2, "Range Table"="", "Read Callback"="", "Write Callback"="", "Supported Models"="", "Instrument Options"="", "Flags"=0, "Help"="Inverts the screenshot colors.\n\nAvailable Repeated Capabilities:\nNone\n\nRemote-control command(s):\nPOWer:REPort:INVert"}, {"Level"=3, "Class Only"=TRUE, "Identifier"="", "Descriptive Name"="Content", "Data Type"=0, "Command"="", "Access"=0, "Range Table"="", "Read Callback"="", "Write Callback"="", "Supported Models"="", "Instrument Options"="", "Flags"=0, "Help"="Defines the content of report."}, {"Level"=4, "Class Only"=FALSE, "Identifier"="RSSCOPE_ATTR_POWER_ANALYSIS_REPORT_CONTENT_TITLE", "Descriptive Name"="Power Analysis Report Content Title", "Data Type"=3, "Command"="POW:REP:CONT:TITL", "Access"=2, "Range Table"="", "Read Callback"="", "Write Callback"="", "Supported Models"="", "Instrument Options"="", "Flags"=0, "Help"="Adds a Title page to the report. The contents can be set up in the &apos;DUT&apos;\n\nAvailable Repeated Capabilities:\nNone\n\nRemote-control command(s):\nPOWer:REPort:CONTent:TITLe"}, {"Level"=4, "Class Only"=FALSE, "Identifier"="RSSCOPE_ATTR_POWER_ANALYSIS_REPORT_CONTENT_MSETUP", "Descriptive Name"="Power Analysis Report Content Measurement Setup", "Data Type"=0, "Command"="POW:REP:CONT:MSET", "Access"=2, "Range Table"="RsScope_rngPowerAnalysisReportContentSetup", "Read Callback"="", "Write Callback"="", "Supported Models"="", "Instrument Options"="", "Flags"=0, "Help"="Adds a graphic of the measurement setup.\n\nAvailable Repeated Capabilities:\nNone\n\nRemote-control command(s):\nPOWer:REPort:CONTent:MSETup"}, {"Level"=4, "Class Only"=FALSE, "Identifier"="RSSCOPE_ATTR_POWER_ANALYSIS_REPORT_CONTENT_SETTINGS", "Descriptive Name"="Power Analysis Report Content Settings", "Data Type"=0, "Command"="POW:REP:CONT:SETT", "Access"=2, "Range Table"="RsScope_rngPowerAnalysisReportContentSetup", "Read Callback"="", "Write Callback"="", "Supported Models"="", "Instrument Options"="", "Flags"=0, "Help"="Adds the settings of the analysis.\n\nAvailable Repeated Capabilities:\nNone\n\nRemote-control command(s):\nPOWer:REPort:CONTent:SETTings"}, {"Level"=4, "Class Only"=FALSE, "Identifier"="RSSCOPE_ATTR_POWER_ANALYSIS_REPORT_CONTENT_VSETUP", "Descriptive Name"="Power Analysis Report Content Vertical Setup", "Data Type"=0, "Command"="POW:REP:CONT:VSET", "Access"=2, "Range Table"="RsScope_rngPowerAnalysisReportContentSetup", "Read Callback"="", "Write Callback"="", "Supported Models"="", "Instrument Options"="", "Flags"=0, "Help"="Adds the vertical setup settings.\n\nAvailable Repeated Capabilities:\nNone\n\nRemote-control command(s):\nPOWer:REPort:CONTent:VSETup"}, {"Level"=4, "Class Only"=FALSE, "Identifier"="RSSCOPE_ATTR_POWER_ANALYSIS_REPORT_CONTENT_HSETUP", "Descriptive Name"="Power Analysis Report Content Horizontal Setup", "Data Type"=0, "Command"="POW:REP:CONT:HSET", "Access"=2, "Range Table"="RsScope_rngPowerAnalysisReportContentSetup", "Read Callback"="", "Write Callback"="", "Supported Models"="", "Instrument Options"="", "Flags"=0, "Help"="Adds the horizontal setup settings.\n\nAvailable Repeated Capabilities:\nNone\n\nRemote-control command(s):\nPOWer:REPort:CONTent:HSETup"}, {"Level"=4, "Class Only"=FALSE, "Identifier"="RSSCOPE_ATTR_POWER_ANALYSIS_REPORT_CONTENT_TSETUP", "Descriptive Name"="Power Analysis Report Content Trigger Setup", "Data Type"=0, "Command"="POW:REP:CONT:TSET", "Access"=2, "Range Table"="RsScope_rngPowerAnalysisReportContentSetup", "Read Callback"="", "Write Callback"="", "Supported Models"="", "Instrument Options"="", "Flags"=0, "Help"="Adds the trigger setup settings.\n\nAvailable Repeated Capabilities:\nNone\n\nRemote-control command(s):\nPOWer:REPort:CONTent:TSETup"}, {"Level"=4, "Class Only"=FALSE, "Identifier"="RSSCOPE_ATTR_POWER_ANALYSIS_REPORT_CONTENT_MEAS", "Descriptive Name"="Power Analysis Report Content Measured Signal", "Data Type"=0, "Command"="POW:REP:CONT:MSIG", "Access"=2, "Range Table"="RsScope_rngPowerAnalysisReportContentSetup", "Read Callback"="", "Write Callback"="", "Supported Models"="", "Instrument Options"="", "Flags"=0, "Help"="Adds a diagram of the measured signal.\n\nAvailable Repeated Capabilities:\nNone\n\nRemote-control command(s):\nPOWer:REPort:CONTent:MSIGnal"}, {"Level"=4, "Class Only"=FALSE, "Identifier"="RSSCOPE_ATTR_POWER_ANALYSIS_REPORT_CONTENT_RESULTS", "Descriptive Name"="Power Analysis Report Content Results", "Data Type"=0, "Command"="POW:REP:CONT:RESU", "Access"=2, "Range Table"="RsScope_rngPowerAnalysisReportContentSetup", "Read Callback"="", "Write Callback"="", "Supported Models"="", "Instrument Options"="", "Flags"=0, "Help"="Adds the result box.\n\nAvailable Repeated Capabilities:\nNone\n\nRemote-control command(s):\nPOWer:REPort:CONTent:RESU"}, {"Level"=2, "Class Only"=TRUE, "Identifier"="", "Descriptive Name"="Power Quality", "Data Type"=0, "Command"="", "Access"=0, "Range Table"="", "Read Callback"="", "Write Callback"="", "Supported Models"="", "Instrument Options"="", "Flags"=0, "Help"="The &apos;Power Quality&apos; analysis measurements include the real power, the reactive power and the apparent power as well as the power factor. The crest factors and the phase angle between the current and voltage are also measured. These properties describe the power transfer in the system and allow you to characterize the power quality of the system."}, {"Level"=3, "Class Only"=FALSE, "Identifier"="RSSCOPE_ATTR_START_POWER_QUALITY_MEASUREMENT", "Descriptive Name"="Start Power Quality Measurement", "Data Type"=4, "Command"="POW:QUAL:EXEC", "Access"=1, "Range Table"="", "Read Callback"="", "Write Callback"="", "Supported Models"="", "Instrument Options"="", "Flags"=0, "Help"="Starts the power quality measurement.\n\nAvailable Repeated Capabilities:\nNone\n\nRemote-control command(s):\nPOWer:QUALity:EXECute"}, {"Level"=3, "Class Only"=FALSE, "Identifier"="RSSCOPE_ATTR_POWER_QUALITY_FREQUENCY", "Descriptive Name"="Power Quality Frequency", "Data Type"=0, "Command"="POW:QUAL:FREQ", "Access"=2, "Range Table"="RsScope_rngPowerQualityFrequency", "Read Callback"="", "Write Callback"="", "Supported Models"="", "Instrument Options"="", "Flags"=0, "Help"="Sets the input frequency of the source signal in Hz.\n\nAvailable Repeated Capabilities:\nNone\n\nRemote-control command(s):\nPOWer:QUALity:FREQ"}, {"Level"=3, "Class Only"=FALSE, "Identifier"="RSSCOPE_ATTR_POWER_QUALITY_CUSTOM_FREQUENCY", "Descriptive Name"="Power Quality Custom Frequency", "Data Type"=1, "Command"="POW:QUAL:FCUS", 
